vi "Pre Launch Init.vi"(11 "Task_Abstr in":refnum<class "Task_Abstr.lvclass">) -> (0 "error out":errorcluster, 3 "Task_Abstr out":refnum<class "Task_Abstr.lvclass">)   [LabVIEW 2025, in "Task_Abstr.lvlib" / "Task_Abstr.lvclass"]
doc: "<p>(<strong>Filename</strong>: <span class=\"dnl\">Actor Framework.lvlib:Actor.lvclass:Pre Launch Init.vi</span>)</p>\n<p>Defines behavior that occurs after the <a href=\"nihelplauncher://docs/csh?context=lvcore_lvcomm_af_launch_nested_actor\">Launch Nested Actor</a> method is invoked but before the actor's Actor Core method begins running.</p>\n<p>By default, this method does nothing. A descendant class may override it to define behavior.</p>"
uses:
  Task_Abstr.lvclass
  DataContainer.ctl
  WaveformData.ctl
  Task_Abstr.lvclass/Task_Abstr.ctl
  <vilib>/ActorFramework/Actor/Actor.lvclass
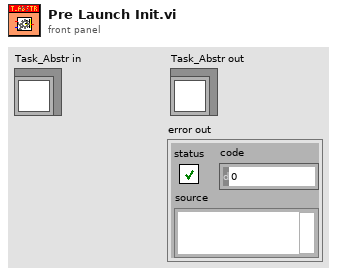
[diagram p1: front panel]
types:
  T1 = typedef "Task_Abstr.lvlib/Task_Abstr.lvclass/DataContainer.ctl" = map{string, T2}
  T2 = typedef "Task_Abstr.lvlib/Task_Abstr.lvclass/WaveformData.ctl" = cluster{"StartTime":timestamp, "StopTime":timestamp, "Waveform":waveform(dbl)[]}
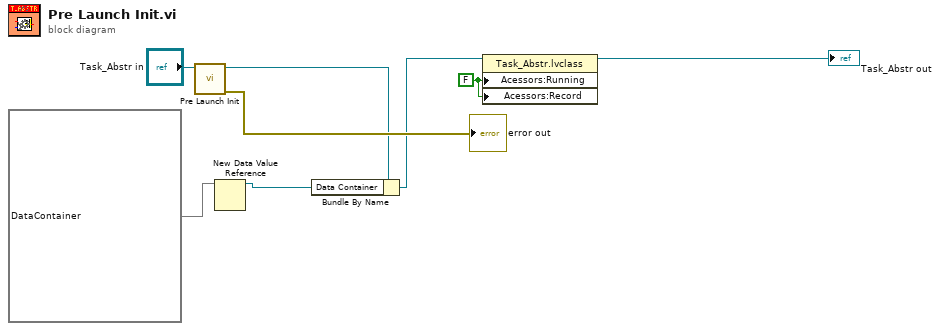
[diagram p0: block diagram]
diagram:
  w1 = FALSE ("Running")
  n1 = call-parent "Pre Launch Init.vi"("Actor in"="Task_Abstr in") -> ("error out"=→"error out":errorcluster, "Actor out"=w5:refnum<class "Task_Abstr.lvclass">)  [unwired: 9 in]
  n2 = New Data Value Reference(data value=T1 {} ("map")) -> (data value reference=w4:refnum<data-value>)  [unwired: 1 in, 1 out]
  n3 = Bundle By Name(cluster=w5, "Data Container"=w4) -> (w3:refnum<class "Task_Abstr.lvclass">)
  n4 = property class="Task_Abstr.lvclass"(reference=w3, "Acessors:Running"=w1, "Acessors:Record"=w1) -> (reference out=→"Task_Abstr out":refnum<class "Task_Abstr.lvclass">)  [unwired: 1 in, 1 out]
